vi "readSensors.vi"(0 "SPI Configs In":T4, 1 "IMU Config In":T1={"Accelerometer Bias"=[0, 0, 0], "Accelerometer Scale"=0, "Gyro Bias"=[0, 0, 0], "Gyro Scale"=0}, 2 "Motor Torque":fxp<+/-,32,16>) -> (3 "Motor Data Out":T2, 4 "Encoder Data Out":T6, 5 "IMU1 Data Out":T5, 6 "IMU2 Data Out":T5)   [LabVIEW 2019]
uses:
  SPI/SPI Config.ctl
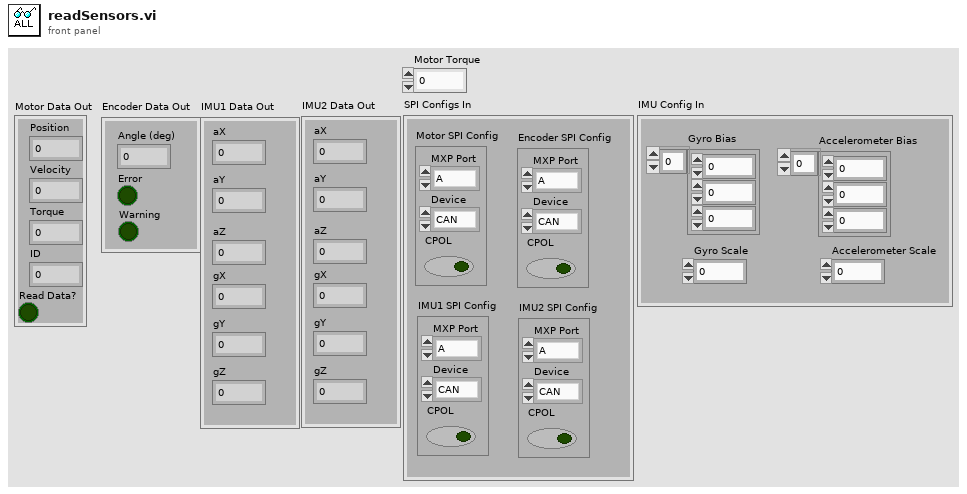
[diagram p1: front panel]
types:
  T1 = cluster{"Accelerometer Bias":i16[], "Accelerometer Scale":i16, "Gyro Bias":i16[], "Gyro Scale":i16}
  T2 = cluster{"Position":fxp<+/-,32,16>, "Velocity":fxp<+/-,32,16>, "Torque":fxp<+/-,32,16>, "ID":u32, "Read Data?":bool}
  T3 = typedef "SPI Config.ctl" = cluster{"MXP Port":enum16{"A", "B"}, "Device":enum16{"CAN", "ENC", "IMU1", "IMU2"}, "CPOL":bool}
  T4 = cluster{"Motor SPI Config":T3, "Encoder SPI Config":T3, "IMU1 SPI Config":T3, "IMU2 SPI Config":T3}
  T5 = cluster{fxp<+/-,32,16>, fxp<+/-,32,16>, fxp<+/-,32,16>, fxp<+/-,32,16>, fxp<+/-,32,16>, fxp<+/-,32,16>}
  T6 = cluster{"Angle (deg)":fxp<+,32,16>, "Error":bool, "Warning":bool}
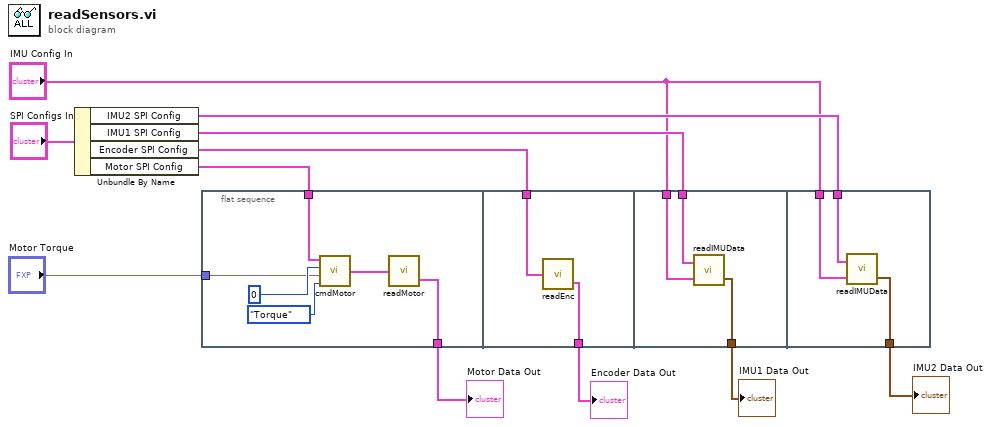
[diagram p0: block diagram]
diagram:
  n1 = Unbundle By Name("SPI Configs In") -> ("IMU2 SPI Config"=w3:T3, "IMU1 SPI Config"=w4:T3, "Encoder SPI Config"=w5:T3, "Motor SPI Config"=w6:T3)
  n2 = flat-sequence {
    tunnel: [w16] -> w2
    tunnel: "Motor Torque" -> [w13]
    tunnel: w6 -> [w12]
    tunnel: [w19] -> w11
    tunnel: w5 -> [w18]
    tunnel: [w22] -> w10
    tunnel: w4 -> [w21]
    tunnel: "IMU Config In" -> [w20]
    tunnel: [w25] -> w9
    tunnel: w3 -> [w24]
    tunnel: "IMU Config In" -> [w23]
    frame #0 {
      n3 = call "cmdMotor.vi"("Mode"=enum16{"Position", "Velocity", "Torque"}."Torque", "Control Value"=w13, "ID"=u32 0, "SPI Config In"=w12) -> ("SPI Config Out"=w17:T3)
      n4 = call "readMotor.vi"("SPI Config In"=w17) -> ("Data Out"=w16:T2)  [unwired: 1 out]
    }
    frame #1 {
      n5 = call "readEnc.vi"("SPI Config In"=w18) -> ("Data Out"=w19:T6)  [unwired: 1 out]
    }
    frame #2 {
      n6 = call "readIMUData.vi"("IMU Config In"=w20, "SPI Config In"=w21) -> ("Data Out"=w22:T5)  [unwired: 1 out]
    }
    frame #3 {
      n7 = call "readIMUData.vi"("IMU Config In"=w23, "SPI Config In"=w24) -> ("Data Out"=w25:T5)  [unwired: 1 out]
    }
  }
  "Encoder Data Out" <- w11
  "IMU1 Data Out" <- w10
  "IMU2 Data Out" <- w9
  "Motor Data Out" <- w2
